vi "Ballard XML Generator.Core Configuration.vi"(11 "string in":string) -> (3 "string out":string)   [LabVIEW 2020]
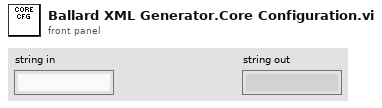
[diagram p1: front panel]
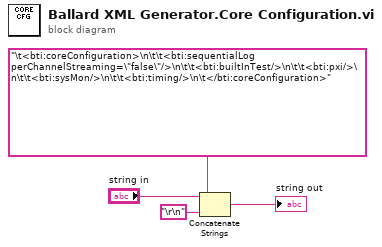
[diagram p0: block diagram]
diagram:
  n1 = Concatenate Strings("string in", "\t<bti:coreConfiguration>\n\t\t<bti:sequentialLog perChannelStreaming=\"false\"/>\n\t\t<bti:builtInTest/>\n\t\t<bti:pxi/>\n\t\t<bti:sysMon/>\n\t\t<bti:timing/>\n\t</bti:coreConfiguration>" ("string"), "\r\n") -> (→"string out":string)
